vi "Actuator Point 2 Array.vi"(1 "Actuator Point":T1) -> (0 "Array":dbl[](array[numeric]))   [LabVIEW 2013]
uses:
  Metadata/Actuator Point.ctl
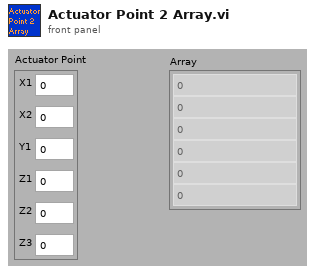
[diagram p1: front panel]
types:
  T1 = typedef "Actuator Point.ctl" = cluster{"X1":dbl, "X2":dbl, "Y1":dbl, "Z1":dbl, "Z2":dbl, "Z3":dbl}
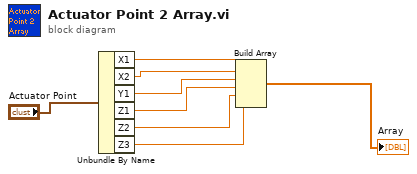
[diagram p0: block diagram]
diagram:
  n1 = Unbundle By Name("Actuator Point") -> ("X1"=w2:dbl, "X2"=w3:dbl, "Y1"=w4:dbl, "Z1"=w5:dbl, "Z2"=w6:dbl, "Z3"=w7:dbl)
  n2 = Build Array(w2, w3, w4, w5, w6, w7) -> (→"Array":dbl[])
